vi "POST (Buffer).vi"(6 "timeout":i32=10000, 7 "output file":path, 8 "error in":errorcluster, 9 "buffer":string, 10 "url":string, 11 "http-method in":refnum<class "net-http-client.lvclass">) -> (0 "error out":errorcluster, 2 "response":refnum<class "response.lvclass">, 3 "http-method out":refnum<class "net-http-client.lvclass">)   [LabVIEW 2020, in "net-http-client.lvclass"]
uses:
  net-http-client.lvclass
  net-http-client.lvclass/net-http-client.ctl
  <vilib>/Viviota/Viviota HTTP Client NET/Types/method_enum.ctl
  <vilib>/Viviota/Viviota HTTP Client NET/HttpClient_NET.lvlib
  net-response/net-response.lvclass
  <vilib>/Viviota/Viviota HTTP Client NET/LabVIEWHTTPClient_NET/HttpClient_NET.lvclass
  classes/response/response.lvclass
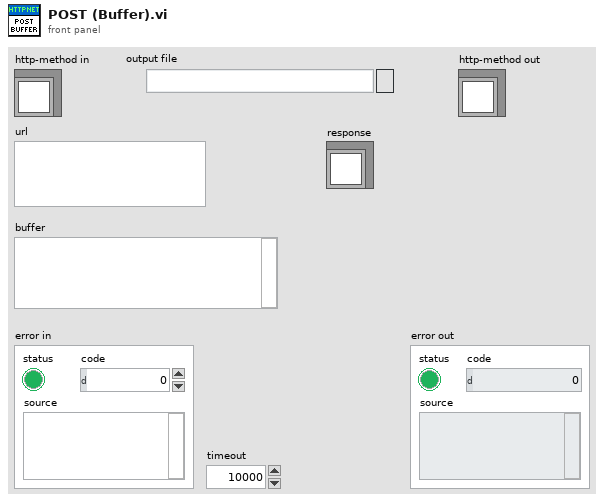
[diagram p1: front panel]
types:
  T1 = typedef "HttpClient_NET.lvlib/method_enum.ctl" = enum16{"GET", "PUT", "POST", "DELETE", "HEAD", "TRACE", "SEND"}
  T2 = typedef "HttpClient_NET.lvlib/ResponseHeaders_Cluster.ctl" = cluster{"ResponseHeader":refnum<class "HttpHeaders_Response.lvclass">, "ContentHeaders":refnum<class "HttpHeaders_Content.lvclass">}
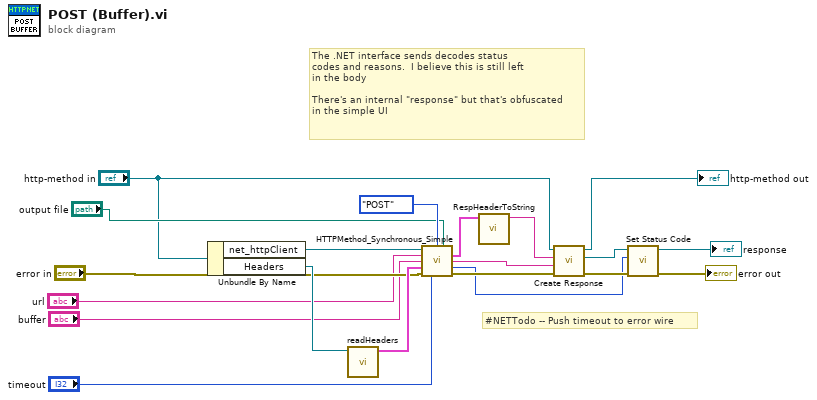
[diagram p0: block diagram]
diagram:
  # "#NETTodo -- Push timeout to error wire"
  # "The .NET interface sends decodes status\ncodes and reasons.  I believe this is still left\nin the body\n\nThere's an internal \"response\" but that's obfuscated\nin the simple UI"
  n1 = Unbundle By Name("http-method in") -> ("net_httpClient"=w19:refnum<class "HttpClient_NET.lvclass">, "Headers"=w11:refnum<data-value>)
  n2 = call "readHeaders.vi"("HeaderRef In"=w11) -> ("Headers"=w10:cluster{"key":string, "value":string}[])  [unwired: 10 in]
  n3 = call <vilib>:"HTTPMethod_Synchronous_Simple.vi"("LabVIEWHTTPClient_NET in"=w19, "Method"=method_enum."POST", "output file"="output file", "URL"="url", "buffer"="buffer", "request headers"=w10, "error in (no error)"="error in", "Timeout_ms (10000)"="timeout") -> ("Headers"=w16:T2, "Response"=w17:string, "StatusCode"=w12:i32, "error out"=w18:errorcluster)  [unwired: 1 in, 3 out]
  n4 = call "RespHeaderToString.vi"("Headers"=w16) -> ("HeaderString"=w15:string)  [unwired: 10 in]
  n5 = call-dynamic "Create Response.vi"("error in (no error)"=w18, "body"=w17, "headers"=w15, "http-client"="http-method in") -> ("error out"=w13:errorcluster, "response"=w14:refnum<class "response.lvclass">, "http-client out"=→"http-method out":refnum<class "net-http-client.lvclass">)  [unwired: 5 in]
  n6 = call "Set Status Code.vi"("error in (no error)"=w13, "StatusCode"=w12, "net-response in"=w14) -> ("error out"=→"error out":errorcluster, "net-response out"=→"response":refnum<class "response.lvclass">)  [unwired: 7 in]
